vi "Read Host to Target FIFO.vi"(8 "error in (no error)":errorcluster) -> (0 "error out":errorcluster, 3 "Host to Target FIFO":u64[](array[numeric]))   [LabVIEW 2016]
uses:
  Host/Typedefs/IO Buffer Operation.ctl
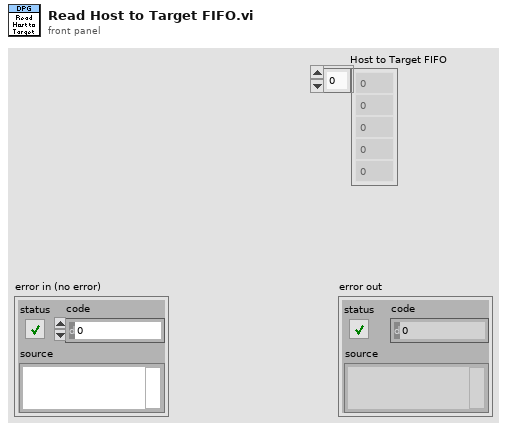
[diagram p1: front panel]
types:
  T1 = typedef "IO Buffer Operation.ctl" = enum16{"Initialize", "Write IO Data_Rd", "Read IO Data_Rd", "Write IO Data_Wr", "Read IO Data_Wr", "Write  IO Data_Dir", "Read  IO Data_Dir", "Write Host to Target FIFO", "Read Host to Target FIFO", "Write Target to Host FIFO", "Read Target to Host FIFO", "Write Monitor Enable?", "Read Monitor Enable?", "Close"}
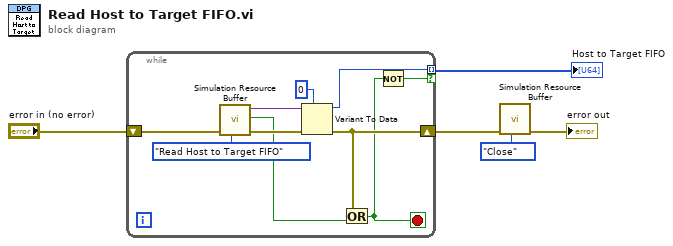
[diagram p0: block diagram]
diagram:
  n1 = while {
    tunnel: [w12] -> w5 mode=indexing if=w9
    shift-right: [w8] -> w4
    shift-left: "error in (no error)" -> [w11]
    stop <- w6 stop-if-true
    n2 = call "Simulation Resource Buffer.vi"("IO Buffer Operation"=IO_Buffer_Operation."Read Host to Target FIFO", "error in (no error)"=w11) -> ("error out"=w14:errorcluster, "Timed Out?"=w7:bool, "Data out"=w13:variant)  [unwired: 7 in]
    n3 = Variant To Data(error in=w14, type=u64 0 ("Target to Host Data"), Variant=w13) -> (data=w12:u64, error out=w8:errorcluster)
    n4 = Or(x=w8, y=w7) -> (x .or. y?=w6:bool)
    n5 = Not(x=w6) -> (.not. x?=w9:bool)
  }
  "Host to Target FIFO" <- w5
  n6 = call "Simulation Resource Buffer.vi"("IO Buffer Operation"=IO_Buffer_Operation."Close", "error in (no error)"=w4) -> ("error out"=→"error out":errorcluster)  [unwired: 7 in, 2 out]
